vi "IND560 Serial Tester.vi"(7 "Use While Loop?":bool, 8 "Error In":errorcluster, 11 "VISA Input":refnum<visa-resource-name>) -> (0 "Error Out":errorcluster, 3 "Net Weight":dbl)   [LabVIEW 2018]
panel:
  out "IND560 Serial Data":string[][](array[string])
  in  "stop":bool
  out "Loop Number":i32
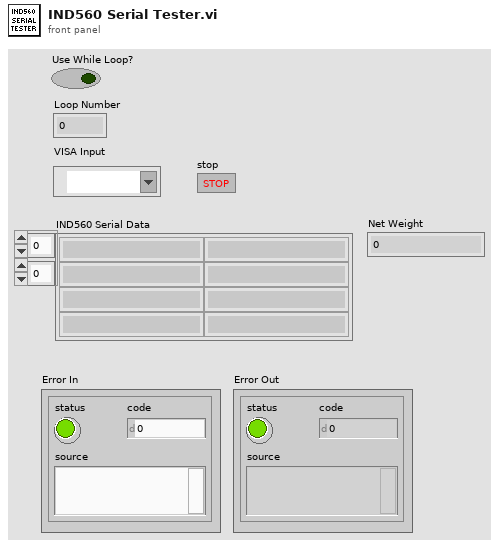
[diagram p1: front panel]
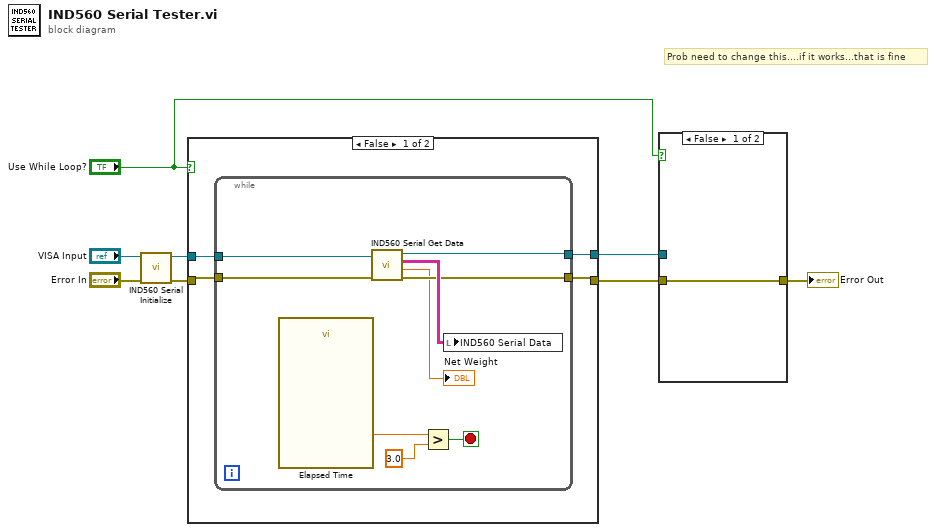
[diagram p0: block diagram]
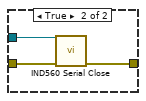
[diagram p2: hidden frame]
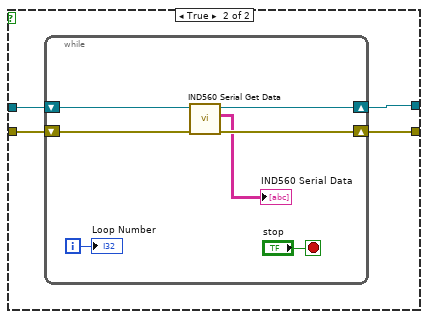
[diagram p3: hidden frame]
diagram:
  # "Prob need to change this....if it works...that is fine"
  n1 = call "IND560 Serial Initialize.vi"("Error In"="Error In", "VISA Refnum in"="VISA Input") -> ("Error Out"=w8:errorcluster, "VISA Refnum Out"=w7:refnum<visa-resource-name>)  [unwired: 8 in]
  n2 = case shown="False" "Use While Loop?" {
    tunnel: w8 -> [w11 w25]
    tunnel: w7 -> [w12 w24]
    tunnel: [w9 w23] -> w5
    tunnel: [w10 w22] -> w4
    frame False {
      n3 = while {
        tunnel: w12 -> [w20]
        tunnel: w11 -> [w19]
        tunnel: [w18] -> w10
        tunnel: [w17] -> w9
        stop <- w14 stop-if-true
        n4 = call "Elapsed Time"() -> ("Elapsed Time (s)"=w16:dbl)  [unwired: 12 in, 7 out]
        n5 = call "IND560 Serial Get Data.vi"("error in (no error)"=w19, "VISA Refnum in"=w20) -> ("error out"=w18:errorcluster, "Gross Weight"=→"Net Weight":dbl, "IND560 Serial Data"=w21:string[][], "VISA Refnum out"=w17:refnum<visa-resource-name>)  [unwired: 6 in]
        n6 = Greater?(x=w16, y=3.0) -> (0:w14:bool)
        n7 = local write "IND560 Serial Data"(w21) -> ()
      }
    }
    frame True {
      n8 = while {
        shift-right: [w31] -> w23
        shift-left: w24 -> [w28]
        shift-right: [w30] -> w22
        shift-left: w25 -> [w27]
        i -> [w29]
        stop <- "stop" stop-if-true
        n9 = call "IND560 Serial Get Data.vi"("error in (no error)"=w27, "VISA Refnum in"=w28) -> ("error out"=w30:errorcluster, "IND560 Serial Data"=→"IND560 Serial Data":string[][], "VISA Refnum out"=w31:refnum<visa-resource-name>)  [unwired: 6 in, 1 out]
        "Loop Number" <- w29
      }
    }
  }
  n10 = case shown="False" "Use While Loop?" {
    tunnel: w5 -> [_ w36]
    tunnel: w4 -> [w33 w35]
    tunnel: [w33 w34] -> w3
    frame False {
    }
    frame True {
      n11 = call "IND560 Serial Close.vi"("error in (no error)"=w35, "VISA Refnum in"=w36) -> ("error out"=w34:errorcluster)  [unwired: 9 in]
    }
  }
  "Error Out" <- w3
